vi "Z Aux Direct Base And Move Abs.vi"(7 "pfDisancelist":sgl, 8 "error in (no error)":errorcluster caption="错误输入（无错误）", 9 "piAxislist":i32, 10 "imaxaxises":i32, 11 "handle":u32) -> (0 "error out":errorcluster caption="错误输出", 1 "piAxislist out":i32, 2 "function return":i32, 3 "handle out":u32, 5 "pfDisancelist out":sgl)   [LabVIEW 2015, in "zauxdll.lvlib"]
doc: "int32 __stdcall ZAux_Direct_BaseAndMoveAbs(ZMC_HANDLE handle, int imaxaxises, int *piAxislist, float *pfDisancelist);"
uses:
  zauxdll.lvlib
  zauxdll.dll
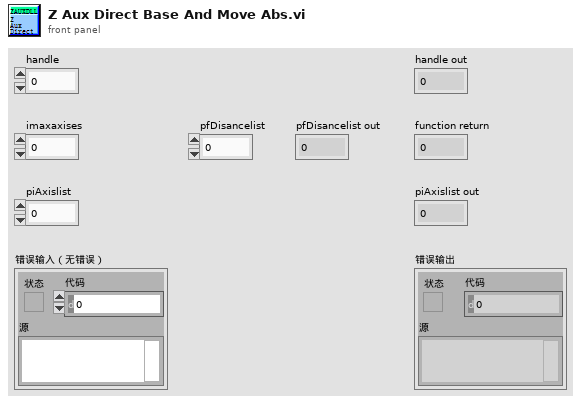
[diagram p1: front panel]
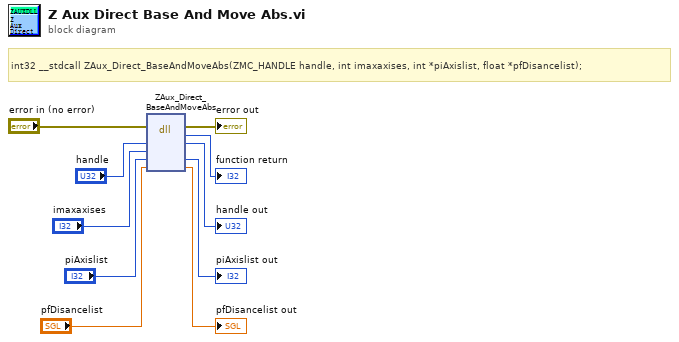
[diagram p0: block diagram]
diagram:
  # "int32 __stdcall ZAux_Direct_BaseAndMoveAbs(ZMC_HANDLE handle, int imaxaxises, int *piAxislist, float *pfDisancelist);"
  n1 = dll-call lib="C:/Users/VIC/Desktop/GOGORO_Oringnal - Panasonic/system/LLB/zmotion/zaux/zauxdll.*" fn="ZAux_Direct_BaseAndMoveAbs"(error in="error in (no error)", "handle"="handle", "imaxaxises"="imaxaxises", "piAxislist"="piAxislist", "pfDisancelist"="pfDisancelist") -> (error out=→"error out":errorcluster, →"function return":i32, "handle"=→"handle out":u32, "piAxislist"=→"piAxislist out":i32, "pfDisancelist"=→"pfDisancelist out":sgl)  [unwired: 3 in, 1 out]
